vi "Progetto SAM - Andrea Alecce.vi"() -> ()   [LabVIEW 2018]
uses:
  <vilib>/sound2/lvsound2.llb/Sound Data Format.ctl
  <vilib>/sound2/lvsound2.llb/Sound Input Read (DBL).vi
  <vilib>/measure/maspectr.llb/FFT Spectrum (Mag-Phase) for N Chan.vi
  <vilib>/Utility/file.llb/Write Delimited Spreadsheet (string).vi
  <vilib>/measure/NI_MAPro.lvlib
panel:
  in  "Chiudi sessione":bool
  in  "Pause Button":bool
  in  "Stop REC":bool
  in  "REC Button":bool
  in  "Canale Sorgente":u32
  in  "sound format":T1={"sample rate (S/s)"=22050.0, "number of channels"=2, "bits per sample"=16}
  in  "Durata acquisizione":dbl=0.2 min=0.1 step=0.1
  in  "Shuntdown Time":i32=-1 min=-1 step=1000
  in  "Soglia":dbl=0.0009999999999999996 step=0.0001
  out "error out":errorcluster
  out "Spettro":cluster{"f0":dbl, "df":dbl, "magnitude":dbl[]}[](graph)
  out "t0":timestamp[](array[timestamp])
  out "Signal":waveform(dbl)[](graph) caption="Waveform Graph"
  in  "db ON":bool
  in  "IIR filter specifications":T2={"Topology"=enum."Butterworth", "Type"=enum."Lowpass", "Order"=1, "Lower Fc"=100.0, "Upper Fc"=200.0, "PB Ripple"=1.0, "SB Attenuation"=60.0} {"PB Ripple" format="%0.2f"; "SB Attenuation" format="%0.2f"; "Lower Fc" format="%0.2p"; "Upper Fc" format="%0.2p"}
  in  "optional IIR filter specifications":T3={"Lower PB"=100.0, "Upper PB"=0.0, "Lower SB"=200.0, "Upper SB"=0.0, "PB Gain"=-3.0, "SB Gain"=-60.0, "Scale"=TRUE} {"PB Gain" format="%0.2f"; "SB Gain" format="%0.2f"; "Lower SB" format="%0.2p"; "Upper SB" format="%0.2f"; "Lower PB" format="%0.2p"; "Upper PB" format="%0.2f"}
  out "IIR ON":bool
  out "FIR ON":bool
  in  "?":bool
  in  "optional FIR specifications":T4={"PB Gain"=-3.0, "SB Gain"=-60.0, "Scale"=TRUE, "Window"=enum."Flat Top"} {"SB Gain" format="%.2p"; "PB Gain" format="%.2p"}
  in  "FIR filter specifications":T5={"Topology"=enum."Off", "Type"=enum."Lowpass", "#Taps"=50, "Lower PB"=100.0, "Upper PB"=0.0, "Lower SB"=200.0, "Upper SB"=0.0} {"Lower SB" format="%0.2p"; "Upper SB" format="%0.2p"; "Lower PB" format="%0.2p"; "Upper PB" format="%0.2p"}
  out "new file path (Not A Path if cancelled)":path
  out "appended path":path
  out "n° chunck":i32
  out "Freq ad ampiezza max":string
  out "Ampiezza min":string
  out "Freq ad ampiezza min":string
  out "Ampiezza max":string
  out "Evento Audio":bool
  out "PAUSE TIME":timestamp[](array[timestamp])
  out "STOP Time":timestamp[](array[timestamp])
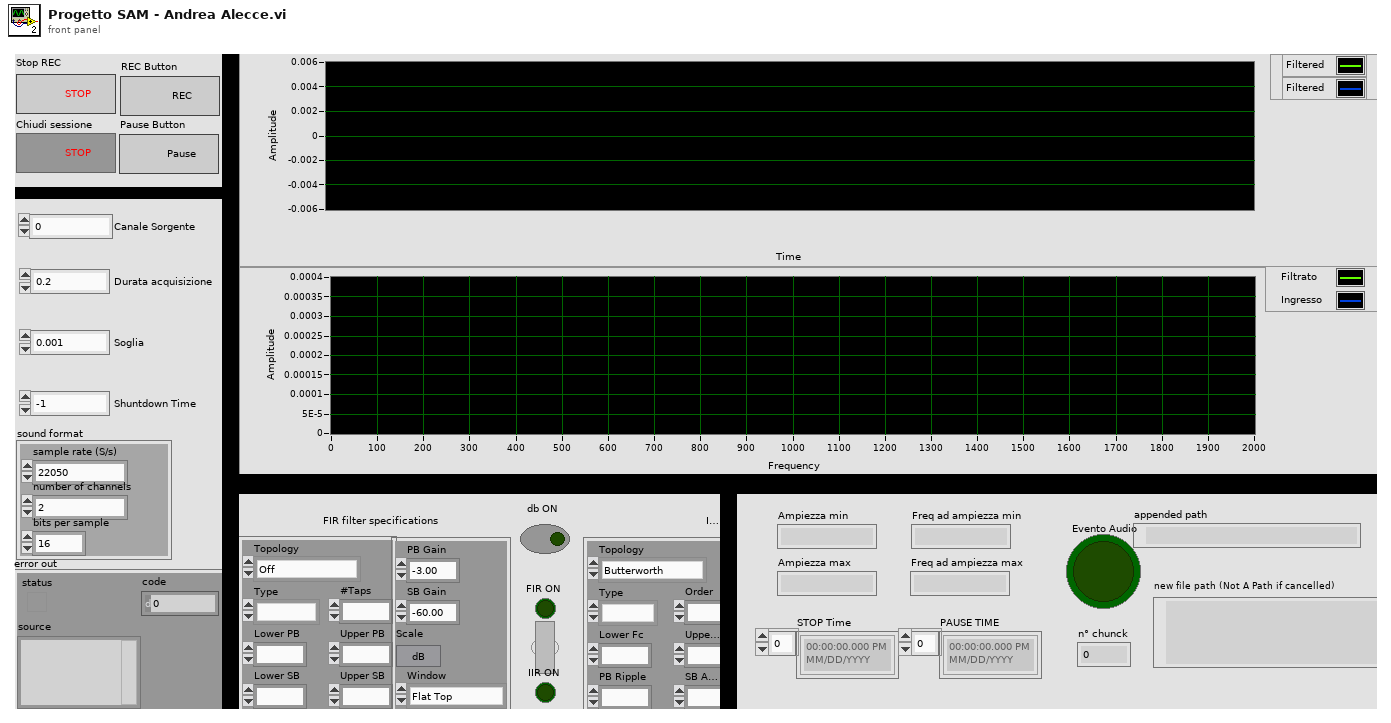
[diagram p1: front panel]
types:
  T1 = typedef "Sound Data Format.ctl" = cluster{"sample rate (S/s)":dbl, "number of channels":i32, "bits per sample":i32}
  T2 = cluster{"Topology":enum16{"Off", "Butterworth", "Chebyshev", "Inverse Chebyshev", "Elliptic", "Bessel"}, "Type":enum16{"Lowpass", "Highpass", "Bandpass", "Bandstop"}, "Order":i32, "Lower Fc":dbl, "Upper Fc":dbl, "PB Ripple":dbl, "SB Attenuation":dbl}
  T3 = cluster{"Lower PB":dbl, "Upper PB":dbl, "Lower SB":dbl, "Upper SB":dbl, "PB Gain":dbl, "SB Gain":dbl, "Scale":bool}
  T4 = cluster{"PB Gain":dbl, "SB Gain":dbl, "Scale":bool, "Window":enum16{"None", "Hanning", "Hamming", "Triangular", "Blackman", "Exact Blackman", "Blackman-Harris", "Kaiser-Bessel", "Flat Top"}}
  T5 = cluster{"Topology":enum16{"Off", "FIR by Specification", "Equi-ripple FIR", "Windowed FIR"}, "Type":enum16{"Lowpass", "Highpass", "Bandpass", "Bandstop"}, "#Taps":i32, "Lower PB":dbl, "Upper PB":dbl, "Lower SB":dbl, "Upper SB":dbl}
  T6 = cluster{"dB On (F)":bool, "unwrap phase (F)":bool, "convert to degree (F)":bool}
  T7 = typedef "Sound Input Task ID.ctl" = u32
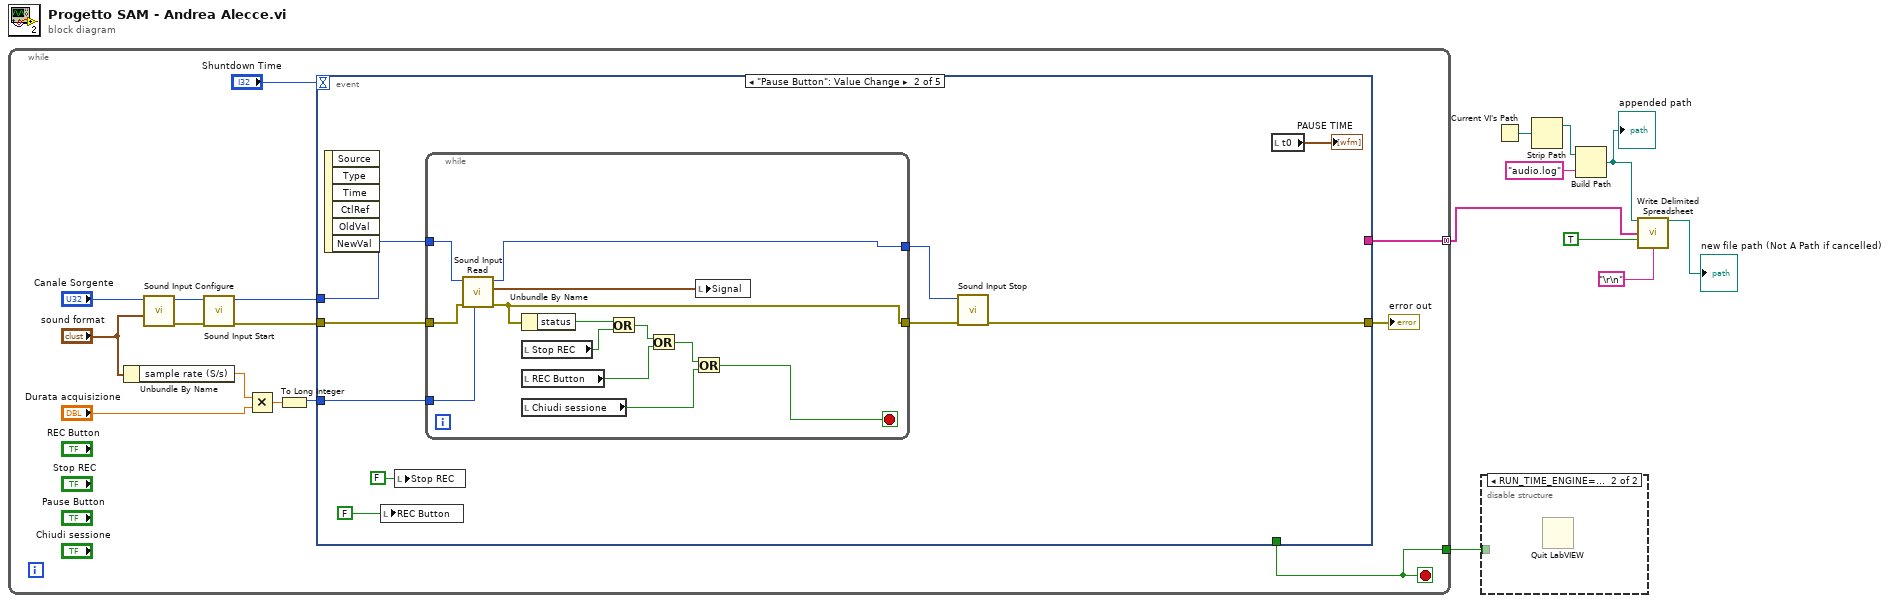
[diagram p0: block diagram]
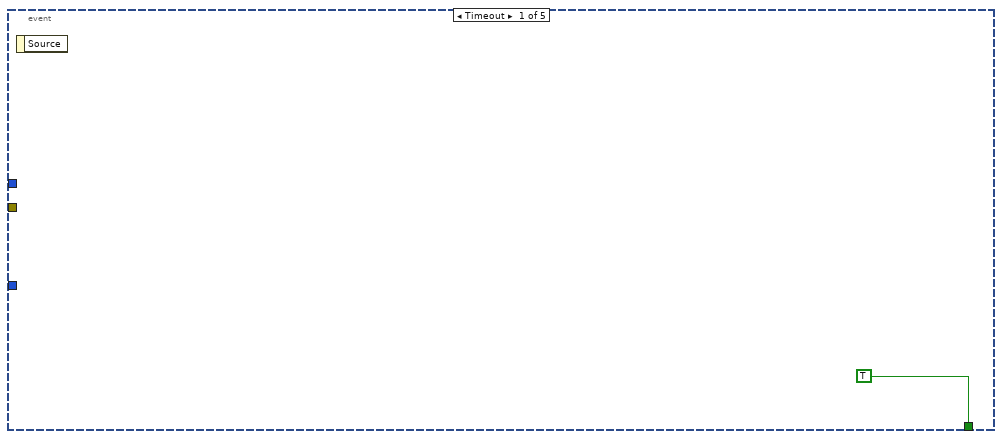
[diagram p3: hidden frame]
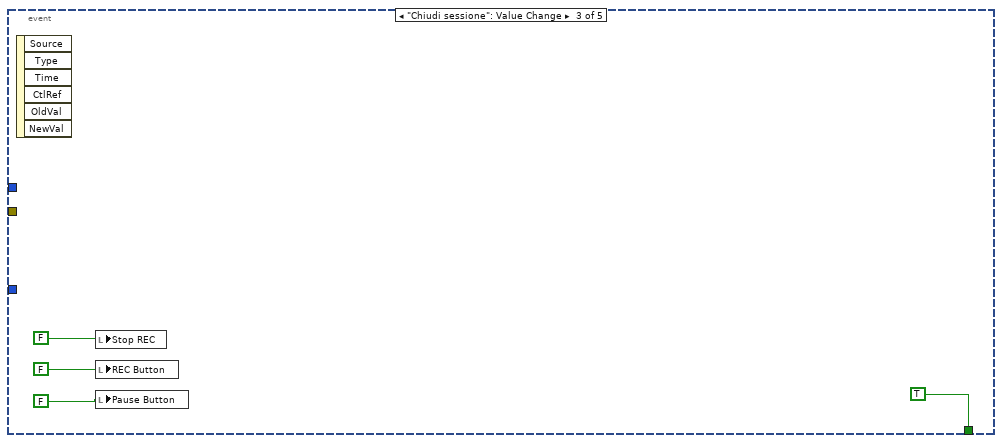
[diagram p4: hidden frame]
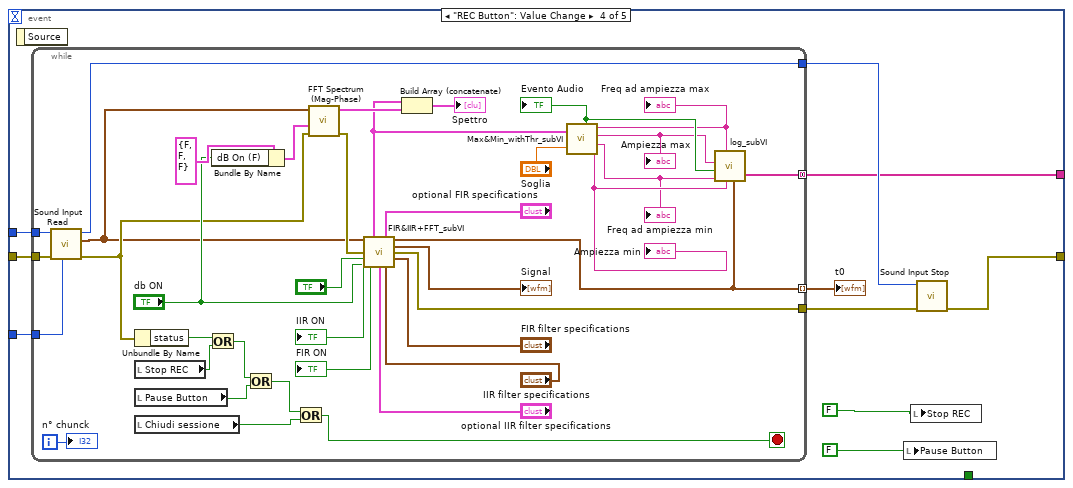
[diagram p5: hidden frame]
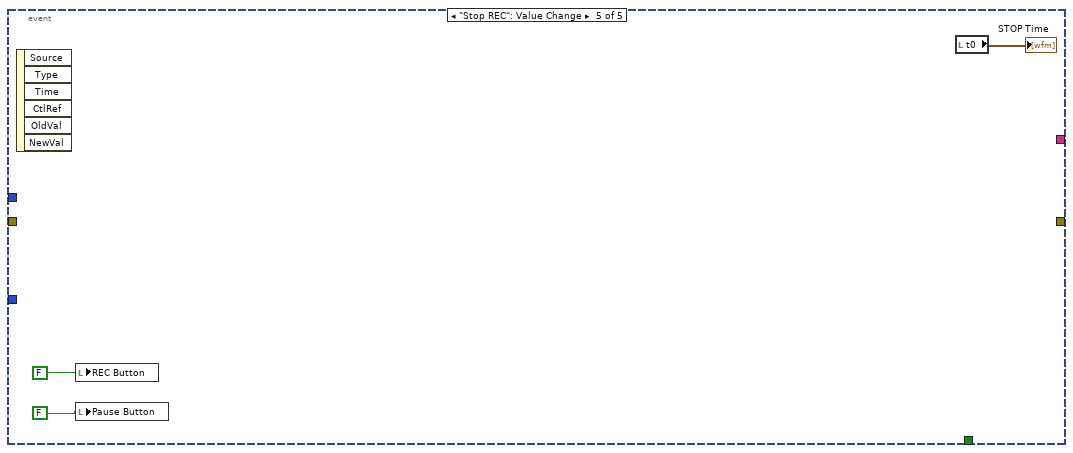
[diagram p6: hidden frame]
diagram:
  n1 = while {
    tunnel: [w12] -> w9
    tunnel: [w11] -> w5 mode=concatenating
    stop <- w12 stop-if-true
    n2 = Unbundle By Name("sound format") -> ("sample rate (S/s)"=w19:dbl)
    n3 = call <vilib>:"Sound Input Configure.vi"("sound format"="sound format", "device ID"="Canale Sorgente") -> ("error out"=w22:errorcluster, "task ID"=w23:T7)  [unwired: 8 in]
    n4 = call <vilib>:"Sound Input Start.vi"("error in (no error)"=w22, "task ID"=w23) -> ("error out"=w15:errorcluster, "task ID out"=w14:T7)  [unwired: 8 in]
    n5 = Multiply(x=w19, y="Durata acquisizione") -> (x*y=w17:dbl)
    n6 = To Long Integer(number=w17) -> (32bit integer=w16:i32)
    n7 = event shown="[1] \"Pause Button\": Value Change" {
      selector: _ -> [_ _ _ _ _]
      dyn-events: _ -> [_ _ _ _ _]
      timeout: "Shuntdown Time" -> [_ _ _ _ _]
      tunnel: [TRUE _ TRUE _ _] -> w12
      tunnel: w16 -> [_ w30 _ w60 _]
      tunnel: w15 -> [_ w26 _ w59 _]
      tunnel: w14 -> [_ w28 _ w58 _]
      tunnel: [_ w31 _ w55 _] -> w13
      tunnel: [_ _ _ w53 _] -> w11
      event Timeout {
        n8 = event-data() -> ()  [unwired: 1 in, 1 out]
      }
      event "Pause Button": Value Change {
        n9 = event-data() -> ()  [unwired: 1 in, 6 out]
        n10 = local write "REC Button"(FALSE ("Record Button")) -> ()
        n11 = local write "Stop REC"(FALSE ("Stop REC")) -> ()
        n12 = while {
          tunnel: w30 -> [w38]
          tunnel: [w37] -> w29
          tunnel: w28 -> [w36]
          tunnel: [w35] -> w27
          tunnel: w26 -> [w34]
          stop <- w39 stop-if-true
          n13 = call-poly <vilib>:"Sound Input Read.vi"("number of samples/ch"=w38, "error in (no error)"=w34, "task ID"=w36) -> ("error out"=w35:errorcluster, "data"=w46:waveform(dbl)[], "task ID out"=w37:T7)  [unwired: 6 in]
          n14 = Unbundle By Name(w35) -> ("status"=w45:bool)
          n15 = local read "Stop REC"() -> (w44:bool)
          n16 = local read "REC Button"() -> (w42:bool)
          n17 = local read "Chiudi sessione"() -> (w40:bool)
          n18 = Or(x=w45, y=w44) -> (x .or. y?=w43:bool)
          n19 = Or(x=w43, y=w42) -> (x .or. y?=w41:bool)
          n20 = Or(x=w41, y=w40) -> (x .or. y?=w39:bool)
          n21 = local write "Signal"(w46) -> ()
        }
        n22 = call <vilib>:"Sound Input Stop.vi"("error in (no error)"=w27, "task ID"=w29) -> ("error out"=w31:errorcluster)  [unwired: 8 in, 1 out]
        n23 = local read "t0"() -> (→"PAUSE TIME":timestamp[])
      }
      event "Chiudi sessione": Value Change {
        n24 = event-data() -> ()  [unwired: 1 in, 6 out]
        n25 = local write "Stop REC"(FALSE ("Pause Button")) -> ()
        n26 = local write "REC Button"(FALSE ("Record Button")) -> ()
        n27 = local write "Pause Button"(FALSE ("Stop REC")) -> ()
      }
      event "REC Button": Value Change {
        n28 = event-data() -> ()  [unwired: 1 in, 1 out]
        n29 = while {
          tunnel: [w98] -> w56
          tunnel: [w72] -> w57
          tunnel: [w79] -> w54 mode=indexing
          tunnel: w60 -> [w95]
          tunnel: w59 -> [w94]
          tunnel: w58 -> [w93]
          tunnel: [w80] -> w53 mode=concatenating
          i -> [w92]
          stop <- w91 stop-if-true
          n30 = call-poly <vilib>:"Sound Input Read.vi"("number of samples/ch"=w95, "error in (no error)"=w94, "task ID"=w93) -> ("error out"=w74:errorcluster, "data"=w61:waveform(dbl)[], "task ID out"=w98:T7)  [unwired: 6 in]
          n31 = Unbundle By Name(w74) -> ("status"=w97:bool)
          n32 = local read "Stop REC"() -> (w64:bool)
          n33 = local read "Pause Button"() -> (w63:bool)
          n34 = local read "Chiudi sessione"() -> (w62:bool)
          n35 = Or(x=w97, y=w64) -> (x .or. y?=w96:bool)
          n36 = Bundle By Name(cluster=T6 {"dB On (F)"=FALSE, "unwrap phase (F)"=FALSE, "convert to degree (F)"=FALSE} ("view"), "dB On (F)"="db ON") -> (w76:T6)
          n37 = Or(x=w96, y=w63) -> (x .or. y?=w90:bool)
          n38 = Or(x=w90, y=w62) -> (x .or. y?=w91:bool)
          n39 = call-poly <vilib>:"FFT Spectrum (Mag-Phase).vi"("error in (no error)"=w74, "view"=w76, "time signals"=w61) -> ("error out"=w73:errorcluster, "magnitudes"=w75:cluster{"f0":dbl, "df":dbl, "magnitude":dbl[]}[])  [unwired: 4 in, 3 out]
          n40 = call "FIR&IIR+FFT_subVI.vi"("waveform array IN"=w61, "optional FIR filter specifications"="optional FIR specifications", "error in (no error)"=w73, "FIR / IIR"="?", "FIR filter specifications"="FIR filter specifications", "db ON"="db ON", "optional IIR filter specifications"="optional IIR filter specifications", "IIR filter specifications"="IIR filter specifications") -> ("magnitude"=w71:cluster{"f0":dbl, "df":dbl, "magnitude":dbl[]}, "t0"=w79:timestamp, "FIR ON"=→"FIR ON":bool, "Signal"=→"Signal":waveform(dbl)[], "error out"=w72:errorcluster, "IIR ON"=→"IIR ON":bool)  [unwired: 2 in]
          n41 = Build Array (concatenate)(w71, w75) -> (→"Spettro":cluster{"f0":dbl, "df":dbl, "magnitude":dbl[]}[])
          n42 = call "Max&Min_withThr_subVI.vi"("Soglia"="Soglia", "magnitude"=w71) -> ("Ampiezza min"=w69:string, "freq ad ampiezza min"=w67:string, "Ampiezza max"=w65:string, "freq ad ampiezza max"=w66:string, "OverThr"=w68:bool)
          "Evento Audio" <- w68
          "Ampiezza min" <- w69
          "Ampiezza max" <- w65
          "Freq ad ampiezza min" <- w67
          "Freq ad ampiezza max" <- w66
          n43 = call "log_subVI.vi"("Ampiezza Min"=w69, "freq ad ampiezza max"=w66, "freq ad ampiezza min"=w67, "Boolean 2"=w68, "Ampiezza Max"=w65, "time stamp"=w79) -> ("Formatted String Output"=w80:string[])  [unwired: 1 in]
          "n° chunck" <- w92
        }
        "t0" <- w54
        n44 = local write "Pause Button"(FALSE ("Stop REC")) -> ()
        n45 = local write "Stop REC"(FALSE ("Pause Button")) -> ()
        n46 = call <vilib>:"Sound Input Stop.vi"("error in (no error)"=w57, "task ID"=w56) -> ("error out"=w55:errorcluster)  [unwired: 8 in, 1 out]
      }
      event "Stop REC": Value Change {
        n47 = event-data() -> ()  [unwired: 1 in, 6 out]
        n48 = local write "REC Button"(FALSE ("Record Button")) -> ()
        n49 = local write "Pause Button"(FALSE ("Pause Button")) -> ()
        n50 = local read "t0"() -> (→"STOP Time":timestamp[])
      }
    }
    "error out" <- w13
  }
  n51 = disable-structure shown="RUN_TIME_ENGINE==True" {
    disable-tunnel: w9 -> [_ _]
    frame condition #0 (active) {
    }
    frame condition #1 {
      n52 = Quit LabVIEW() -> ()  [unwired: 1 in]
    }
  }
  n53 = Current VI's Path() -> (path=w8:path)
  n54 = Strip Path(path=w8) -> (stripped path=w7:path)  [unwired: 1 out]
  n55 = Build Path(base path=w7, name or relative path="audio.log") -> (appended path=w4:path)
  "appended path" <- w4
  n56 = call-poly <vilib>:"Write Delimited Spreadsheet.vi"("file path (dialog if empty)"=w4, "1D data"=w5, "append to file? (new file:F)"=TRUE, "delimiter (\\t)"="\r\n") -> ("new file path (Not A Path if cancelled)"=→"new file path (Not A Path if cancelled)":path)  [unwired: 10 in, 1 out]
